vi "呈现图片.vi"(8 "error in (no error)":errorcluster caption="错误输入（无错误）", 11 "点 输入":refnum<class "点.lvclass"> caption="DNL_LabVIEW Object in") -> (0 "error out":errorcluster caption="错误输出", 2 "Picture":picture caption="图片", 3 "点 输出":refnum<class "点.lvclass"> caption="DNL_LabVIEW Object out")   [LabVIEW 2011, in "点.lvclass"]
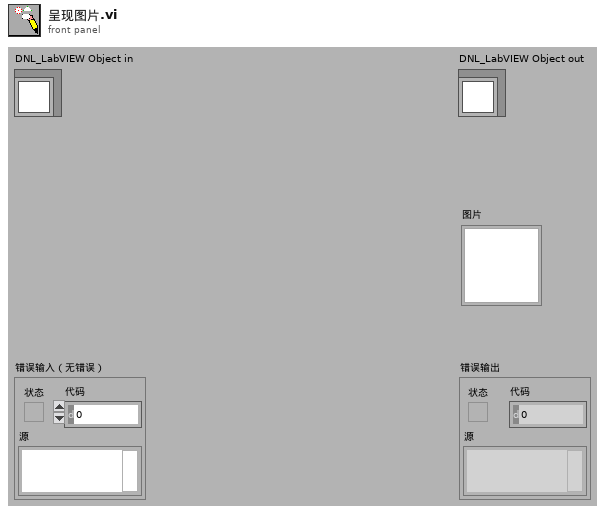
[diagram p1: front panel]
types:
  T1 = typedef "LVPointDoubleTypeDef.ctl" = cluster{"X":dbl, "Y":dbl}
  T2 = cluster{"Width":u16, "Style":enum32{"Solid", "Dash", "Dot", "DashDot", "DashDotDot"}}
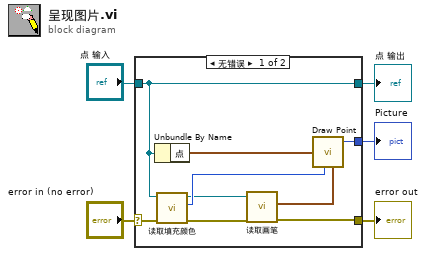
[diagram p0: block diagram]
diagram:
  n1 = case shown="无错误" "error in (no error)" {
    selector: "error in (no error)" -> [w11 w16]
    tunnel: [w8 w16] -> w4
    tunnel: "点 输入" -> [w10 w15]
    tunnel: [w10 w15] -> w2
    tunnel: [w14 _] -> w1
    frame No Error {
      n2 = Unbundle By Name(w10) -> ("点"=w13:T1)
      n3 = call "读取填充颜色.vi"("error in (no error)"=w11, "图形输入"=w10) -> ("error out"=w9:errorcluster, "填充颜色"=w12:u32, "图形输出"=w7:refnum<class "点.lvclass">)  [unwired: 7 in]
      n4 = call "读取画笔.vi"("error in (no error)"=w9, "图形输入"=w7) -> ("error out"=w8:errorcluster, "画笔"=w6:T2)  [unwired: 7 in, 1 out]
      n5 = call <vilib>:"Draw Point.vi"("point(x,y)"=w13, "color(black)"=w12, "pen"=w6) -> ("new picture"=w14:picture)  [unwired: 1 in, 5 out]
    }
    frame Error {
    }
  }
  "error out" <- w4
  "Picture" <- w1
  "点 输出" <- w2
